vi "Add Piece into Wall.vi"(8 "error in (no error)":errorcluster caption="entrée d'erreur (pas d'erreur)", 11 "Game Board en entrée":refnum<class "Game Board.lvclass">) -> (0 "error out":errorcluster caption="sortie d'erreur", 3 "Game Board en sortie":refnum<class "Game Board.lvclass">)   [LabVIEW 2017, in "Game Board.lvclass"]
uses:
  Game Board.lvclass
  Game Board.lvclass/Game Board.ctl
  Wall_class/Wall.lvclass
  Piece of Bricks_class/Piece of Bricks.lvclass
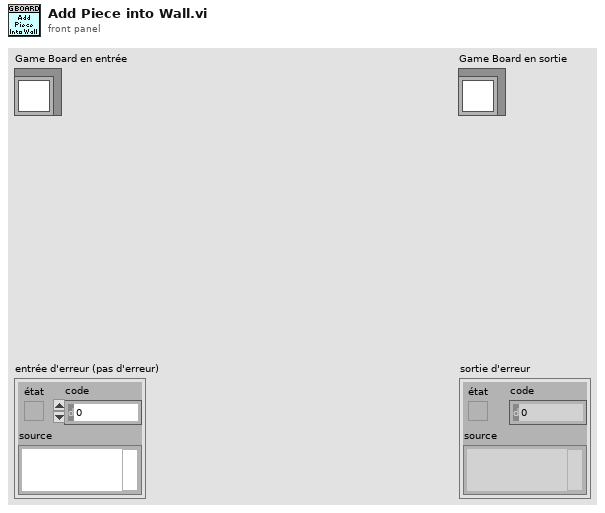
[diagram p1: front panel]
types:
  T1 = typedef "Coordinates.ctl" = cluster{"X":i32, "Y":i32}
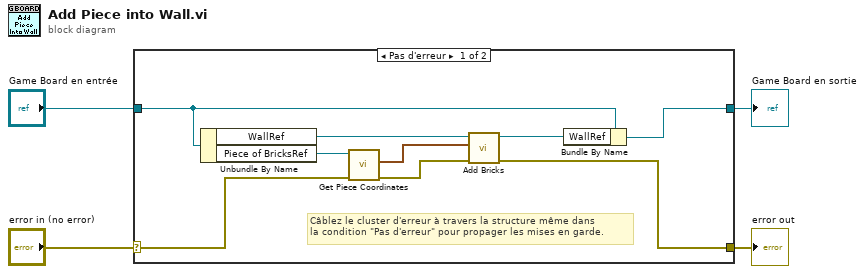
[diagram p0: block diagram]
diagram:
  n1 = case shown="Pas d'erreur" "error in (no error)" {
    selector: "error in (no error)" -> [w5 w15]
    tunnel: [w9 w15] -> w3
    tunnel: [w13 w14] -> w1
    tunnel: "Game Board en entrée" -> [w10 w14]
    frame No Error {
      # "Câblez le cluster d'erreur à travers la structure même dans\nla condition \"Pas d'erreur\" pour propager les mises en garde."
      n2 = Unbundle By Name(w10) -> ("WallRef"=w11:refnum<class "Wall.lvclass">, "Piece of BricksRef"=w8:refnum<class "Piece of Bricks.lvclass">)
      n3 = call-dynamic "Get Piece Coordinates.vi"("error in (no error)"=w5, "object in"=w8) -> ("error out"=w6:errorcluster, "Piece Coordinates"=w7:T1[])  [unwired: 7 in, 1 out]
      n4 = call-dynamic "Add Bricks.vi"("error in (no error)"=w6, "Piece Coordinates"=w7, "object in"=w11) -> ("error out"=w9:errorcluster, "object out"=w12:refnum<class "Wall.lvclass">)  [unwired: 7 in]
      n5 = Bundle By Name(cluster=w10, "WallRef"=w12) -> (w13:refnum<class "Game Board.lvclass">)
    }
    frame Error {
    }
  }
  "error out" <- w3
  "Game Board en sortie" <- w1
